vi "oa_Compute Power Spectrum (1 Channel).vi"(6 "averaging mode":T1(ring), 7 "spectrum settings":cluster{"window type":u32, "block size":i32}={"window type"=1, "block size"=200} {"block size" min=2; "window type" items=["None"=0, "Hanning"=1, "Hamming"=2, "Blackman-Harris"=3, "Exact Blackman"=4, "Blackman"=5, "Flat Top"=6, "4 Term B-Harris"=7, "7 Term B-Harris"=8, "Low Sidelobe"=9, "Gaussian"=62]}, 10 "dr":dbl=1.0 format="%.2p", 11 "Y":dbl[][](array[numeric]) format="%.2f") -> (1 "df":dbl=1.0 format="%.2p", 3 "power spectrum":dbl[][](array[numeric]) format="%.2f")   [LabVIEW 2017, in "SoundVib_Resampling.lvlib"]
uses:
  <vilib>/addons/Sound and Vibration/Order Analysis/Resample Order Tracking/SoundVib_Resampling.lvlib
  <vilib>/Analysis/NI_AALPro.lvlib
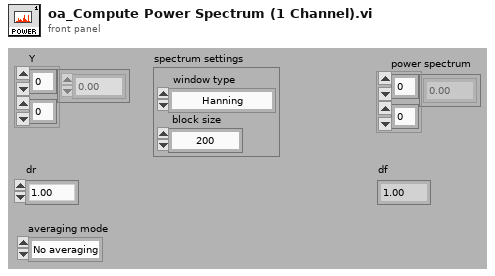
[diagram p1: front panel]
types:
  T1 = enum16{"No averaging", "Vector averaging", "RMS averaging", "Peak hold"}
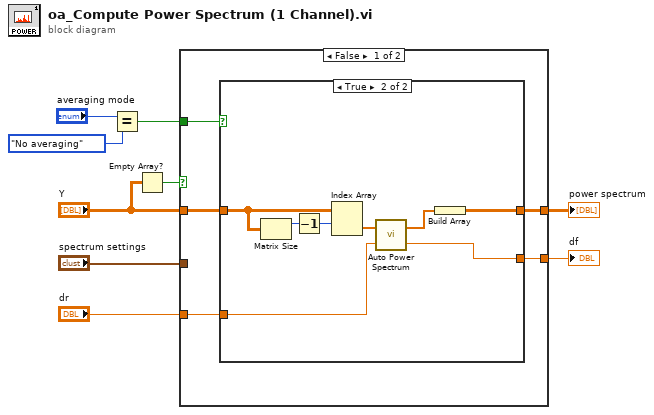
[diagram p0: block diagram]
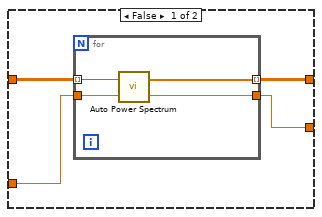
[diagram p2: hidden frame]
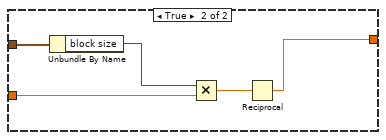
[diagram p3: hidden frame]
diagram:
  n1 = Equal?(x="averaging mode", y=T1."No averaging" ("averaging mode")) -> (x = y?=w7:bool)
  n2 = Empty Array?(array="Y") -> (empty?=w2:bool)
  n3 = case shown="False" w2 {
    tunnel: w7 -> [w14 _]
    tunnel: "dr" -> [w13 w32]
    tunnel: [w12 _] -> w5
    tunnel: [w11 w31] -> w4
    tunnel: "Y" -> [w10 _]
    tunnel: "spectrum settings" -> [_ w35]
    frame False {
      n4 = case shown="True" w14 {
        tunnel: w10 -> [w15 w23]
        tunnel: w13 -> [w17 w28]
        tunnel: [w18 w26] -> w12
        tunnel: [w16 w25] -> w11
        frame False {
          n5 = for {
            tunnel: w15 -> [w22] mode=indexing
            tunnel: [w21] -> w18 mode=indexing
            tunnel: w17 -> [w20]
            tunnel: [w19] -> w16
            n6 = call <vilib>:"Auto Power Spectrum.vi"("dt"=w20, "Signal (V)"=w22) -> ("df"=w19:dbl, "Power Spectrum (V^2 rms)"=w21:dbl[])
          }
        }
        frame True {
          n7 = Matrix Size(0:w23) -> (1:w24:i32)  [unwired: 1 out]
          n8 = Decrement(x=w24) -> (x-1=w30:i32)
          n9 = Index Array(array=w23, index (row)=w30) -> (element=w29:dbl[])  [unwired: 1 in]
          n10 = call <vilib>:"Auto Power Spectrum.vi"("dt"=w28, "Signal (V)"=w29) -> ("df"=w25:dbl, "Power Spectrum (V^2 rms)"=w27:dbl[])
          n11 = Build Array(w27) -> (w26:dbl[][])
        }
      }
    }
    frame True {
      n12 = Unbundle By Name(w35) -> ("block size"=w33:i32)
      n13 = Multiply(x=w33, y=w32) -> (x*y=w34:dbl)
      n14 = Reciprocal(x=w34) -> (1/x=w31:dbl)
    }
  }
  "power spectrum" <- w5
  "df" <- w4
